vi "阈值范围选择子VI.vi"() -> (1 "阈值范围":cluster{"Lower value":sgl, "Upper value":sgl}, 3 "确定执行":bool)   [LabVIEW 2018]
panel:
  in  "取消":bool
  in  "确定":bool
  in  "阈值范围选择":cluster{u8, u8}(slide)={0, 255} scale=0.0..255.0
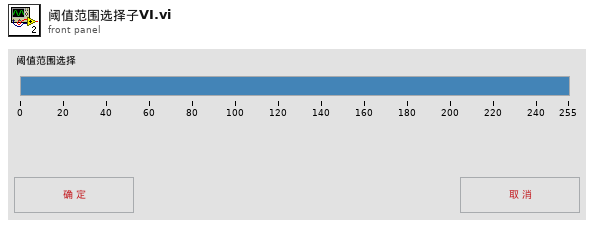
[diagram p1: front panel]
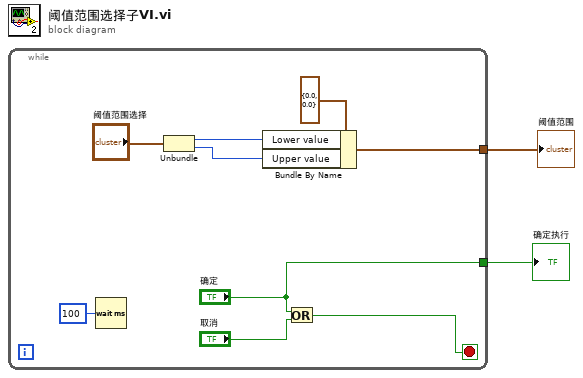
[diagram p0: block diagram]
diagram:
  n1 = while {
    tunnel: [w7] -> w2
    tunnel: ["确定"] -> w1
    stop <- w6 stop-if-true
    n2 = Wait (ms)(milliseconds to wait=u32 100 ("等待时间（毫秒）")) -> ()  [unwired: 1 out]
    n3 = Unbundle("阈值范围选择") -> (w9:u8, w8:u8)
    n4 = Bundle By Name(cluster=cluster{"Lower value":sgl, "Upper value":sgl} {"Lower value"=0.0, "Upper value"=0.0} ("输入簇"), "Lower value"=w9, "Upper value"=w8) -> (w7:cluster{"Lower value":sgl, "Upper value":sgl})
    n5 = Or(x="确定", y="取消") -> (x .or. y?=w6:bool)
  }
  "阈值范围" <- w2
  "确定执行" <- w1
